vi "Set Status with History.vi"(8 "error in (no error)":errorcluster, 10 "Status":string, 11 "Tracker Main.lvlib:Data.lvclass in":refnum<class "Data.lvclass">) -> (0 "error out":errorcluster, 1 "Status History":string[](array[string]), 2 "Status copy":string, 3 "Tracker Main.lvlib:Data.lvclass out":refnum<class "Data.lvclass">)   [LabVIEW 2018, in "Tracker Main.lvlib"]
uses:
  Tracker Main.lvlib
  Data.lvclass
  Data.lvclass/Data.ctl
  Methods/Read Status History.vi
  Methods/Write Status.vi
  Methods/Write Status History.vi
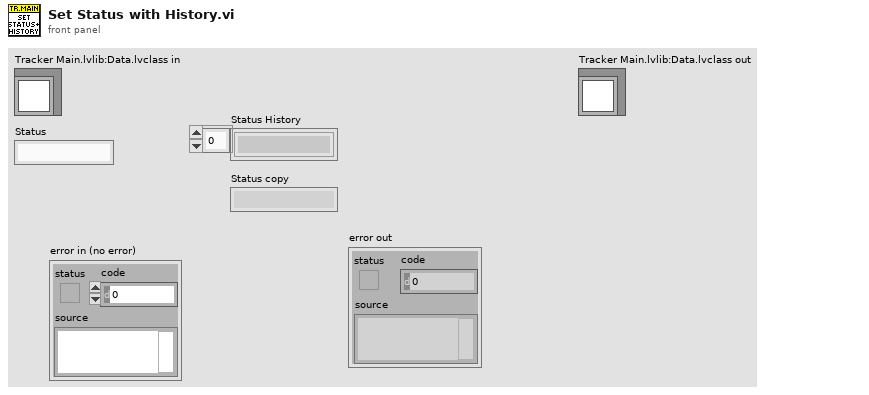
[diagram p1: front panel]
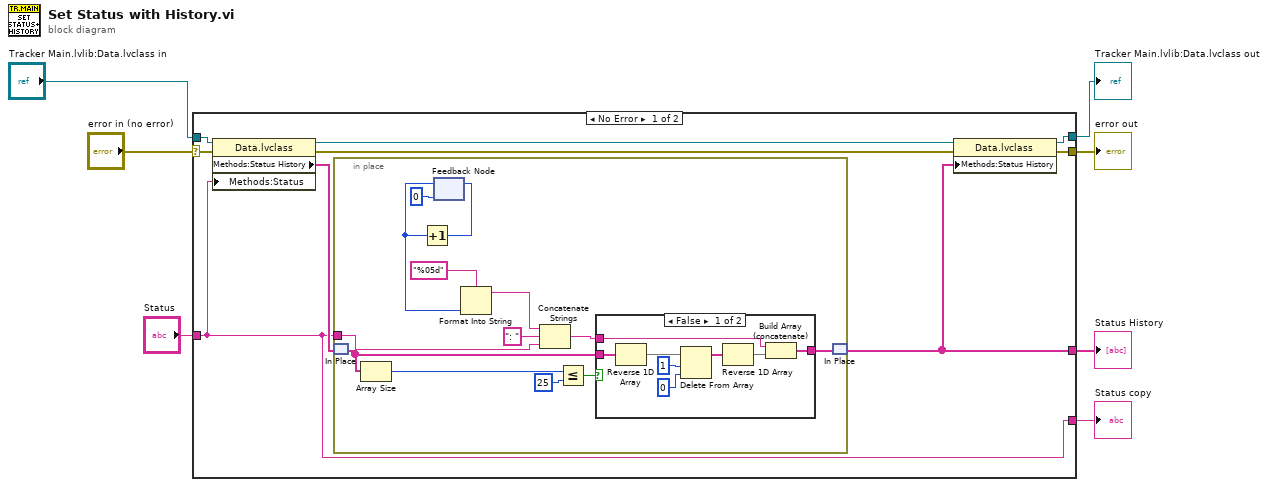
[diagram p0: block diagram]
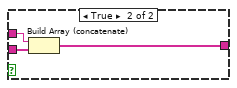
[diagram p2: hidden frame]
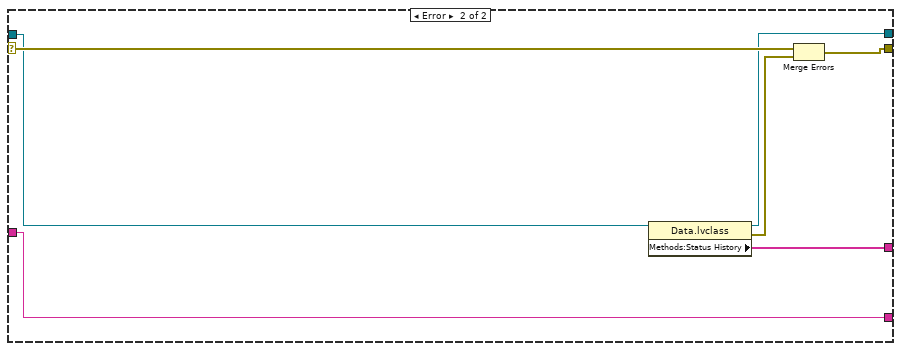
[diagram p3: hidden frame]
diagram:
  n1 = case shown="No Error" "error in (no error)" {
    selector: "error in (no error)" -> [w16 w47]
    tunnel: [w10 w44] -> w6
    tunnel: [w11 w42] -> w5
    tunnel: "Tracker Main.lvlib:Data.lvclass in" -> [w15 w46]
    tunnel: "Status" -> [w8 w41]
    tunnel: [w9 w45] -> w2
    tunnel: [w8 w41] -> w1
    frame No Error {
      n2 = property class="Data.lvclass"(reference=w15, error in=w16, "Methods:Status"=w8) -> (reference out=w13:refnum<class "Data.lvclass">, error out=w12:errorcluster, "Methods:Status History"=w14:string[])
      n3 = in-place {
        in-place-border: w8 -> [w26]
        n4 = in-place-match #1(w14) -> (w18:string[])
        n5 = Array Size(array=w18) -> (size(s)=w29:i32)
        n6 = feedback #2(u32 0) -> (w23:u32)
        n7 = Increment(x=w23) -> (x+1=w24:u32)
        n8 = feedback-in #2(w24) -> ()
        n9 = Format Into String(format string="%05d", w23) -> (resulting string=w20:string)  [unwired: 2 in, 1 out]
        n10 = Concatenate Strings(w20, ": ", w26) -> (w21:string)
        n11 = Less Or Equal?(x=w29, y=25) -> (x <= y?=w27:bool)
        n12 = case shown="False" w27 {
          tunnel: w18 -> [w37 w40]
          tunnel: w21 -> [w31 w39]
          tunnel: [w30 w38] -> w17
          frame False {
            n13 = Reverse 1D Array(array=w37) -> (reversed array=w36:string[])
            n14 = Delete From Array(array=w36, length=1, index=0) -> (array with subset deleted=w33:string[])  [unwired: 1 out]
            n15 = Reverse 1D Array(array=w33) -> (reversed array=w32:string[])
            n16 = Build Array (concatenate)(w31, w32) -> (w30:string[])
          }
          frame True {
            n17 = Build Array (concatenate)(w39, w40) -> (w38:string[])
          }
        }
        n18 = in-place-match #1(w17) -> (w9:string[])
      }
      n19 = property class="Data.lvclass"(reference=w13, error in=w12, "Methods:Status History"=w9) -> (reference out=w11:refnum<class "Data.lvclass">, error out=w10:errorcluster)
    }
    frame Error {
      n20 = property class="Data.lvclass"(reference=w46) -> (reference out=w42:refnum<class "Data.lvclass">, error out=w43:errorcluster, "Methods:Status History"=w45:string[])  [unwired: 1 in]
      n21 = Merge Errors(w47, w43) -> (w44:errorcluster)
    }
  }
  "error out" <- w6
  "Status History" <- w2
  "Status copy" <- w1
  "Tracker Main.lvlib:Data.lvclass out" <- w5
